vi "2 NetVelocity.vi"(8 "Speed 2":dbl, 9 "Angle 2":dbl, 10 "Speed 1":dbl, 11 "Angle 1":dbl) -> (2 "Net Velocity":dbl)   [LabVIEW 2011]
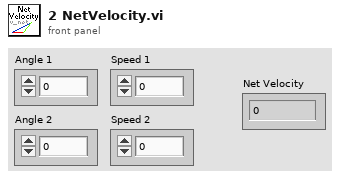
[diagram p1: front panel]
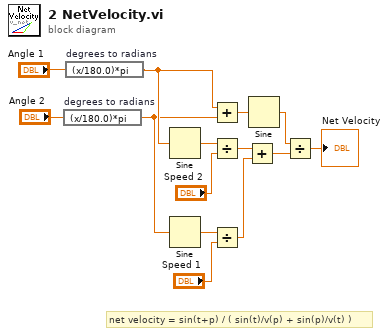
[diagram p0: block diagram]
diagram:
  # "net velocity = sin(t+p) / ( sin(t)/v(p) + sin(p)/v(t) )"
  n1 = expression code="(x/180.0)*pi" "degrees to radians"("Angle 2") -> (w3:dbl)
  n2 = expression code="(x/180.0)*pi" "degrees to radians"("Angle 1") -> (w6:dbl)
  n3 = Sine(x=w6) -> (sin(x)=w10:dbl)
  n4 = Sine(x=w3) -> (sin(x)=w13:dbl)
  n5 = Add(x=w6, y=w3) -> (x+y=w14:dbl)
  n6 = Divide(x=w10, y="Speed 2") -> (x/y=w12:dbl)
  n7 = Divide(x=w13, y="Speed 1") -> (x/y=w11:dbl)
  n8 = Add(x=w12, y=w11) -> (x+y=w8:dbl)
  n9 = Sine(x=w14) -> (sin(x)=w9:dbl)
  n10 = Divide(x=w9, y=w8) -> (x/y=→"Net Velocity":dbl)
